vi "Set_Rel.vi"(0 "VisaCluster":T3, 5 "Range":T2, 7 "Numeric":i32, 9 "Unit":T1, 11 "error in (no error)":errorcluster) -> (4 "VisaCluster":T3, 8 "Answer":string, 15 "error out":errorcluster)   [LabVIEW 2014, in "FH 55.lvlib"]
doc: "Dieses VI setzt den Bezugswert für die Relative-Funktion\n\n\nThis VI sets the reference value for the Relative function"
uses:
  FH 55.lvlib
  TypeDef/VisaCluster.ctl
  TypeDef/Range.ctl
  TypeDef/Unit.ctl
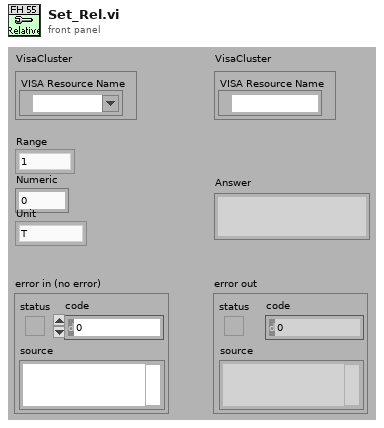
[diagram p1: front panel]
types:
  T1 = typedef "FH 55.lvlib/Unit.ctl" = enum16{"T", "G", "A/m"}
  T2 = typedef "FH 55.lvlib/Range.ctl" = enum16{"1", "2", "3", "4", "5", "6", "7"}
  T3 = typedef "FH 55.lvlib/VisaCluster.ctl" = cluster{"VISA Resource Name":refnum<visa-resource-name>}
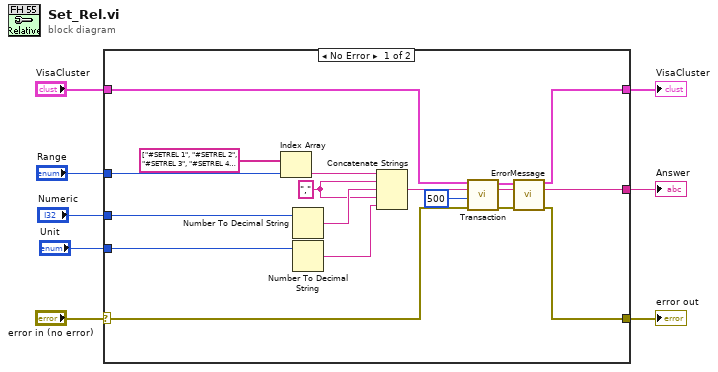
[diagram p0: block diagram]
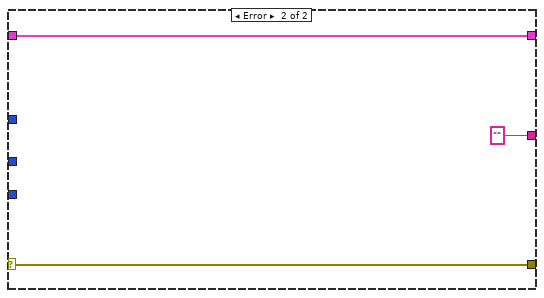
[diagram p2: hidden frame]
diagram:
  n1 = case shown="No Error" "error in (no error)" {
    selector: "error in (no error)" -> [w22 w28]
    tunnel: "VisaCluster" -> [w23 w29]
    tunnel: [w26 w29] -> w4
    tunnel: [w24 w28] -> w6
    tunnel: [w25 ""] -> w5
    tunnel: "Range" -> [w11 _]
    tunnel: "Numeric" -> [w10 _]
    tunnel: "Unit" -> [w9 _]
    frame No Error {
      w16 = ","
      n2 = Index Array(array=string[] ["#SETREL 1", "#SETREL 2", "#SETREL 3", "#SETREL 4", "#SETREL 5", "#SETREL 6", "#SETREL 7", ""], index=w11) -> (element=w13:string)
      n3 = Number To Decimal String(number=w10) -> (decimal integer string=w17:string)  [unwired: 1 in]
      n4 = Number To Decimal String(number=w9) -> (decimal integer string=w15:string)  [unwired: 1 in]
      n5 = Concatenate Strings(w13, w16, w17, w16, w15) -> (w18:string)
      n6 = call "Transaction.vi"("VisaCluster"=w23, "Command"=w18, "Time (150) ms"=u32 500, "error in (no error)"=w22) -> ("VisaCluster"=w19:T3, "Answer"=w20:string, "error out"=w21:errorcluster)  [unwired: 8 in, 1 out]
      n7 = call "ErrorMessage.vi"("VisaCluster"=w19, "Message In"=w20, "error in (no error)"=w21) -> ("VisaCluster"=w26:T3, "Message Out"=w25:string, "error out"=w24:errorcluster)  [unwired: 10 in]
    }
    frame Error {
    }
  }
  "error out" <- w6
  "Answer" <- w5
  "VisaCluster" <- w4
